vi "OriginalTest.vi"() -> ()   [LabVIEW 2010]
uses:
  ROS/Code/SubVIs/_ROSDirection.ctl
  ROS/Code/Console/Servers/ServerSubs/TopicDef.ctl
  ROS/Code/SubVIs/JointMode.ctl
  ROS/Code/SubVIs/BaxterArmsSmall.ctl
  ROS/Code/SubVIs/BaxterSide.ctl
panel:
  in  "Gain":dbl
  in  "Elbow 0 desired angle":dbl
  out "x/y":dbl
  in  "Arm Angles (degrees)":T1
  in  "Mode":T2=1 items=["Position"=1, "Velocity"=2, "Effort"=3]
  in  "Side":T3
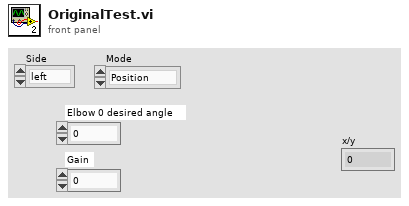
[diagram p1: front panel]
types:
  T1 = typedef "BaxterArmsSmall.ctl" = cluster{"Elbow 0":dbl, "Elbow 1":dbl, "Shoulder 0":dbl, "Shoulder 1":dbl, "Wrist 0":dbl, "Wrist 1":dbl, "Wrist 2":dbl}
  T2 = typedef "JointMode.ctl" = u8
  T3 = typedef "BaxterSide.ctl" = enum16{"left", "right"}
  T4 = typedef "TopicDef.ctl" = cluster{"Topic":string, "Type":string, "Action":T5, "Update (ms)":u16, "write queue":u16}
  T5 = typedef "_ROSDirection.ctl" = enum16{"Node", "Publisher", "Subscriber", "Service Client"}
  T6 = typedef "_ROSControl.ctl" = cluster{"topic port":u16, "Node":string, "topic":string, "type":string, "node port":u32, "error ":errorcluster, "Direction":T5, "APIs":string[], "Update (ms)":u16, "write queue":u16}
  T7 = enum16{"left_e0", "left_e1", "left_s0", "left_s1", "left_w0", "left_w1", "left_w2", "right_e0", "right_e1", "right_s0", "right_s1", "right_w0", "right_w1", "right_w2"}
  T8 = cluster{"Joint Name":string, "Position":dbl, "Velocity":dbl, "Effort":dbl}[]
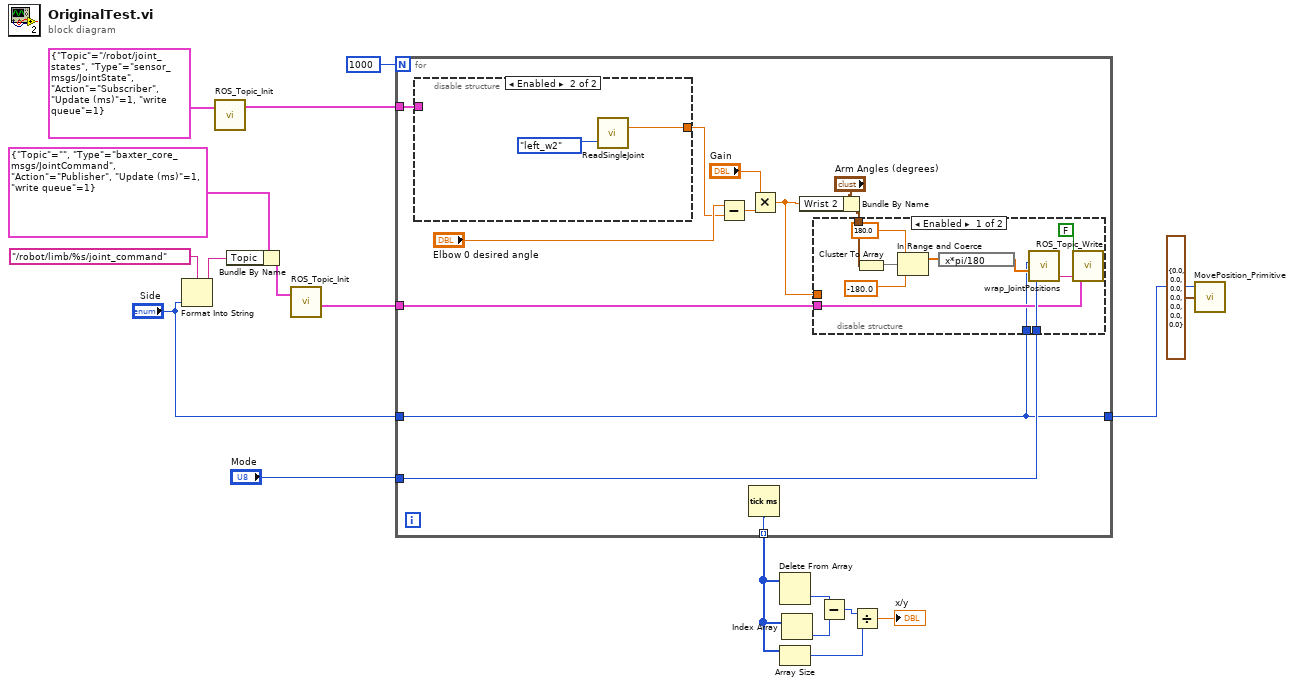
[diagram p0: block diagram]
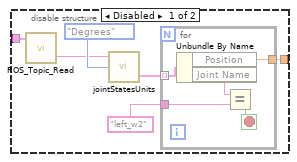
[diagram p2: hidden frame]
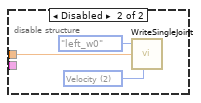
[diagram p3: hidden frame]
diagram:
  n1 = Format Into String(format string="/robot/limb/%s/joint_command" ("Topic"), "Side") -> (resulting string=w16:string)  [unwired: 2 in, 1 out]
  n2 = call "ROS_Topic_Init.vi"("Definitions"=T4 {"Topic"="/robot/joint_states", "Type"="sensor_msgs/JointState", "Action"=enum."Subscriber", "Update (ms)"=1, "write queue"=1}) -> ("ROS out"=w3:T6)  [unwired: 2 in]
  n3 = Bundle By Name(cluster=T4 {"Topic"="", "Type"="baxter_core_msgs/JointCommand", "Action"=enum."Publisher", "Update (ms)"=1, "write queue"=1} ("Definitions"), "Topic"=w16) -> (w14:T4)
  n4 = call "ROS_Topic_Init.vi"("Definitions"=w14) -> ("ROS out"=w4:T6)  [unwired: 2 in]
  n5 = for {
    N: 1000 -> [_]
    tunnel: [w30] -> w9 mode=indexing
    tunnel: "Mode" -> [w29]
    tunnel: "Side" -> [w21]
    tunnel: w4 -> [w27]
    tunnel: w3 -> [w26]
    tunnel: [w21] -> w2
    n6 = disable-structure shown="Enabled" {
      disable-tunnel: w26 -> [w34 _]
      disable-tunnel: [w31 w42] -> w19
      frame Disabled {
        n7 = call "ROS_Topic_Read.vi"("ROS in"=w34) -> ("Reply"=w35:string)  [unwired: 1 in, 1 out]
        n8 = call "jointStatesUnits.vi"("Units (deg)"=enum16{"Radians", "Degrees"}."Degrees", "msg in"=w35) -> ("Joint States"=w32:T8)  [unwired: 1 in, 2 out]
        n9 = for {
          tunnel: w32 -> [w41] mode=indexing
          tunnel: "left_w2" ("Joint Name") -> [w39]
          tunnel: [w37] -> w31
          stop <- w38 stop-if-true
          n10 = Unbundle By Name(w41) -> ("Position"=w37:dbl, "Joint Name"=w40:string)
          n11 = Equal?(x=w40, y=w39) -> (x = y?=w38:bool)
        }
      }
      frame Enabled {
        n12 = call "ReadSingleJoint.vi"("Angle Name"=T7."left_w2") -> ("Position"=w42:dbl)  [unwired: 1 in, 2 out]
      }
    }
    n13 = Subtract(x="Elbow 0 desired angle", y=w19) -> (x-y=w25:dbl)
    n14 = Tick Count (ms)() -> (millisecond timer value=w30:u32)
    n15 = Multiply(x="Gain", y=w25) -> (x*y=w22:dbl)
    n16 = Bundle By Name(cluster="Arm Angles (degrees)", "Wrist 2"=w22) -> (w23:T1)
    n17 = disable-structure shown="Enabled" {
      disable-tunnel: w29 -> [w49 _]
      disable-tunnel: w27 -> [w48 _]
      disable-tunnel: w23 -> [w45 _]
      disable-tunnel: w21 -> [w44 _]
      disable-tunnel: w22 -> [_ w57]
      frame Enabled {
        n18 = Cluster To Array(cluster=w45) -> (array=w54:dbl[])
        n19 = In Range and Coerce(upper limit=180.0 ("Elbow 0"), x=w54, lower limit=-180.0 ("Elbow 0")) -> (coerced(x)=w51:dbl[])  [unwired: 1 out]
        n20 = expression code="x*pi/180"(w51) -> (w50:dbl[])
        n21 = call "wrap_JointPositions.vi"("Mode"=w49, "Positions"=w50, "Side"=w44) -> ("msg out"=w47:string)  [unwired: 3 in]
        n22 = call "ROS_Topic_Write.vi"("Msg in"=w47, "Continuous?"=FALSE, "ROS in"=w48) -> ()  [unwired: 1 in, 1 out]
      }
      frame Disabled {
        w56 = T2 2 items=["Position"=1, "Velocity"=2, "Effort"=3] ("Mode")
        n23 = call "WriteSingleJoint.vi"("Angle Name"=T7."left_w0", "Angle (degrees)"=w57, "Mode"=w56) -> ()  [unwired: 3 in, 1 out]
      }
    }
  }
  n24 = Delete From Array(array=w9) -> (deleted portion=w12:u32)  [unwired: 2 in, 1 out]
  n25 = Array Size(array=w9) -> (size(s)=w8:i32)
  n26 = Index Array(array=w9) -> (element=w11:u32)  [unwired: 1 in]
  n27 = Subtract(x=w12, y=w11) -> (x-y=w10:u32)
  n28 = Divide(x=w10, y=w8) -> (x/y=→"x/y":dbl)
  n29 = call "MovePosition_Primitive.vi"("Side"=w2, "Arm Angles (degrees)"=T1 {"Elbow 0"=0.0, "Elbow 1"=0.0, "Shoulder 0"=0.0, "Shoulder 1"=0.0, "Wrist 0"=0.0, "Wrist 1"=0.0, "Wrist 2"=0.0}) -> ()  [unwired: 4 in, 1 out]
